vi "ShooterBallVelocityCompensation.vi"(2 "Shooter Upper Speed Goal":dbl, 3 "Shooter Lower Speed Goal":dbl) -> (0 "Compensated Upper Speed Goal":dbl, 1 "Compensated Lower Speed Goal":dbl)   [LabVIEW 2020]
uses:
  sensordata.vi
  robotconstants.vi
panel:
  in  "Ball Slip Tuning Parameter":dbl=2.0
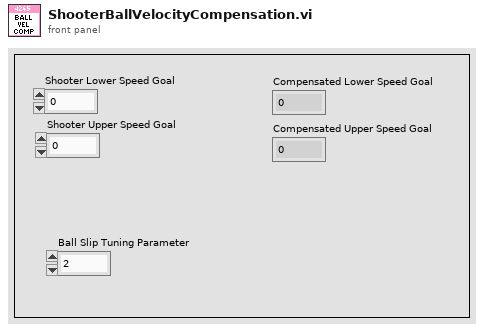
[diagram p1: front panel]
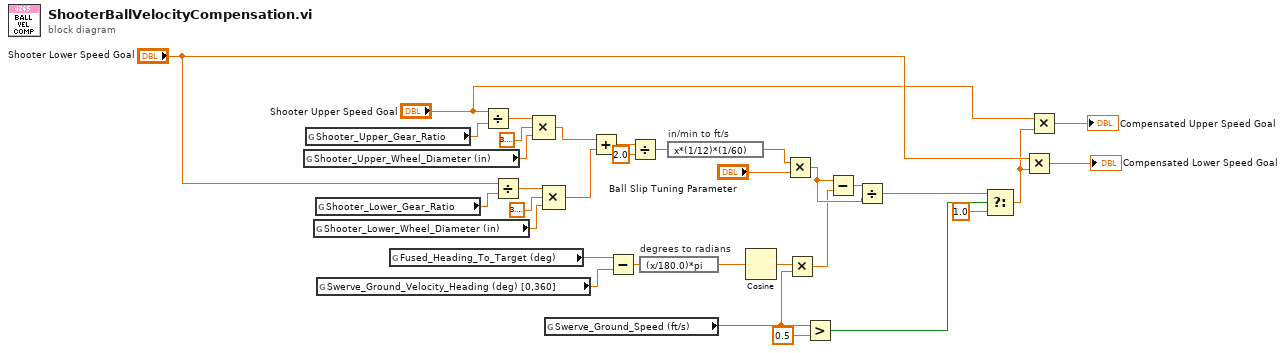
[diagram p0: block diagram]
diagram:
  n1 = global read "robotconstants.vi" "Shooter_Upper_Wheel_Diameter (in)"() -> (w29:dbl)
  n2 = global read "robotconstants.vi" "Shooter_Upper_Gear_Ratio"() -> (w32:dbl)
  n3 = global read "robotconstants.vi" "Shooter_Lower_Wheel_Diameter (in)"() -> (w24:dbl)
  n4 = global read "robotconstants.vi" "Shooter_Lower_Gear_Ratio"() -> (w27:dbl)
  n5 = global read "sensordata.vi" "Swerve_Ground_Velocity_Heading (deg) [0,360]"() -> (w16:dbl)
  n6 = global read "sensordata.vi" "Fused_Heading_To_Target (deg)"() -> (w33:dbl)
  n7 = Divide(x="Shooter Upper Speed Goal", y=w32) -> (x/y=w31:dbl)
  n8 = Divide(x="Shooter Lower Speed Goal", y=w27) -> (x/y=w26:dbl)
  n9 = Compound Arithmetic op=MULTIPLY(w31, 3.141592653589793, w29) -> (w28:dbl)
  n10 = Compound Arithmetic op=MULTIPLY(w26, 3.141592653589793, w24) -> (w23:dbl)
  n11 = global read "sensordata.vi" "Swerve_Ground_Speed (ft/s)"() -> (w11:dbl)
  n12 = Add(x=w28, y=w23) -> (x+y=w22:dbl)
  n13 = Subtract(x=w33, y=w16) -> (x-y=w15:dbl)
  n14 = Divide(x=w22, y=2.0) -> (x/y=w20:dbl)
  n15 = expression code="(x/180.0)*pi" "degrees to radians"(w15) -> (w14:dbl)
  n16 = expression code="x*(1/12)*(1/60)" "in/min to ft/s"(w20) -> (w19:dbl)
  n17 = Cosine(x=w14) -> (cos(x)=w13:dbl)
  n18 = Multiply(x=w19, y="Ball Slip Tuning Parameter") -> (x*y=w17:dbl)
  n19 = Multiply(x=w13, y=w11) -> (x*y=w12:dbl)
  n20 = Greater?(x=w11, y=0.5) -> (0:w9:bool)
  n21 = Subtract(x=w17, y=w12) -> (x-y=w18:dbl)
  n22 = Divide(x=w18, y=w17) -> (x/y=w6:dbl)
  n23 = Select(t=w6, s=w9, f=1.0) -> (s? t:f=w4:dbl)
  n24 = Multiply(x="Shooter Lower Speed Goal", y=w4) -> (x*y=→"Compensated Lower Speed Goal":dbl)
  n25 = Multiply(x="Shooter Upper Speed Goal", y=w4) -> (x*y=→"Compensated Upper Speed Goal":dbl)
